vi "RUSHShoot.vi"(1 "In Cluster":T2) -> (0 "Out Cluster":T1)   [LabVIEW 2012]
panel:
  in  "Speed Multiplier":dbl=0.75
  in  "LinReg Adder":dbl=-0.5
  in  "LinReg Multiplier":dbl=0.01
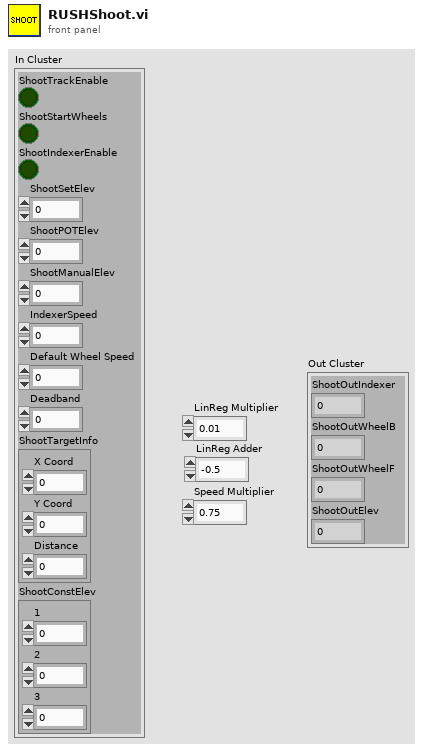
[diagram p1: front panel]
types:
  T1 = cluster{"ShootOutIndexer":dbl, "ShootOutWheelB":dbl, "ShootOutWheelF":dbl, "ShootOutElev":dbl}
  T2 = cluster{"ShootTrackEnable":bool, "ShootStartWheels":bool, "ShootIndexerEnable":bool, "ShootSetElev":dbl, "ShootPOTElev":dbl, "ShootManualElev":dbl, "IndexerSpeed":dbl, "Default Wheel Speed":dbl, "Deadband":dbl, "ShootTargetInfo":cluster{"X Coord":dbl, "Y Coord":dbl, "Distance":dbl}, "ShootConstElev":cluster{"1":dbl, "2":dbl, "3":dbl}}
  T3 = cluster{"X Coord":dbl, "Y Coord":dbl, "Distance":dbl}
  T4 = cluster{"ShootOutIndexer":dbl, "ShootOutWheelB":dbl, "ShootOutWheelF":dbl, "ShootManualElev":dbl}
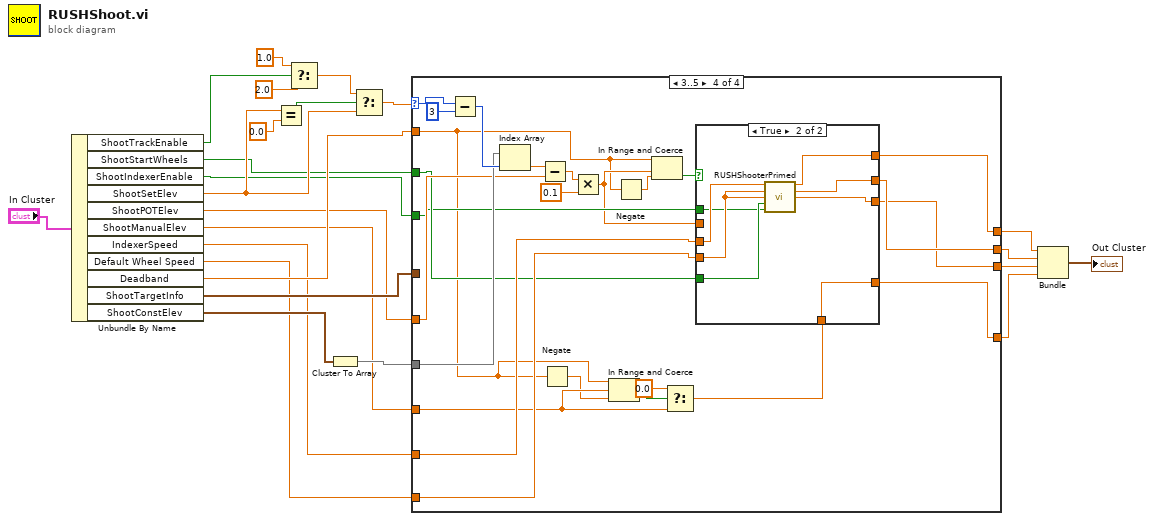
[diagram p0: block diagram]
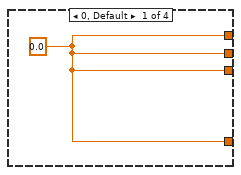
[diagram p2: hidden frame]
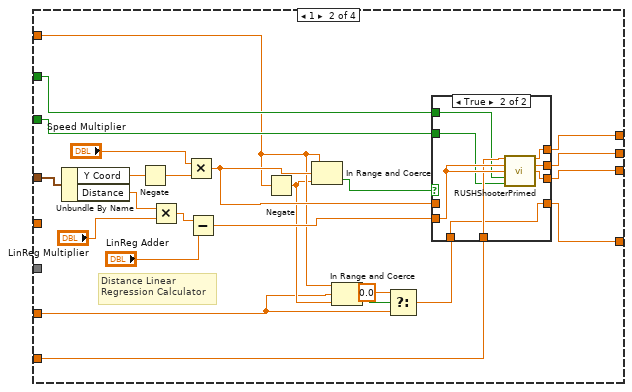
[diagram p3: hidden frame]
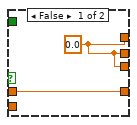
[diagram p4: hidden frame]
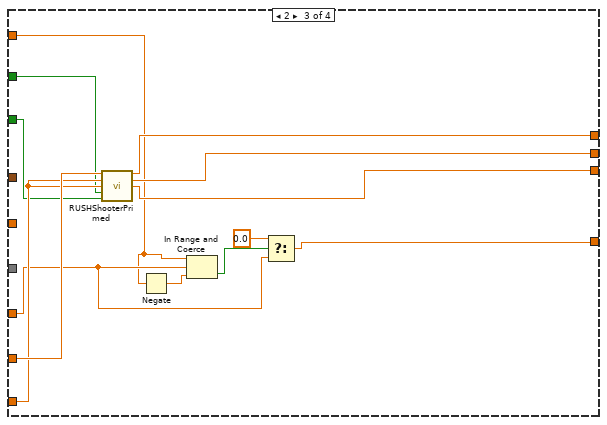
[diagram p5: hidden frame]
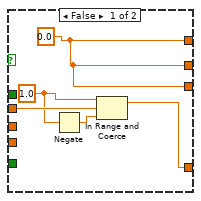
[diagram p6: hidden frame]
diagram:
  n1 = Unbundle By Name("In Cluster") -> ("ShootTrackEnable"=w16:bool, "ShootStartWheels"=w13:bool, "ShootIndexerEnable"=w12:bool, "ShootSetElev"=w15:dbl, "ShootPOTElev"=w10:dbl, "ShootManualElev"=w8:dbl, "IndexerSpeed"=w7:dbl, "Default Wheel Speed"=w6:dbl, "Deadband"=w14:dbl, "ShootTargetInfo"=w11:T3, "ShootConstElev"=w9:cluster{"1":dbl, "2":dbl, "3":dbl})
  n2 = Equal?(x=w15, y=0.0) -> (x = y?=w21:bool)
  n3 = Select(t=1.0, s=w16, f=2.0) -> (s? t:f=w20:dbl)
  n4 = Cluster To Array(cluster=w9) -> (array=w18:dbl[])
  n5 = Select(t=w20, s=w21, f=w15) -> (s? t:f=w19:dbl)
  n6 = case shown="3..5" w19 {
    selector: w19 -> [_ _ _ w97]
    tunnel: w13 -> [_ w44 w70 w83]
    tunnel: w12 -> [_ w43 w69 w82]
    tunnel: w11 -> [_ w49 _ _]
    tunnel: w10 -> [_ _ _ w92]
    tunnel: w18 -> [_ _ _ w94]
    tunnel: w8 -> [_ w27 w63 w75]
    tunnel: [w25 w37 w68 w89] -> w5
    tunnel: [w25 w36 w67 w88] -> w4
    tunnel: [w25 w35 w66 w87] -> w3
    tunnel: [w25 w33 w62 w86] -> w2
    tunnel: w7 -> [_ w32 w72 w85]
    tunnel: w6 -> [_ _ w71 w84]
    tunnel: w14 -> [_ w31 w61 w73]
    frame 0, Default {
      w25 = 0.0 ("ShootOutIndexer")
    }
    frame 1 {
      # "Distance Linear\nRegression Calculator"
      n7 = Unbundle By Name(w49) -> ("Y Coord"=w48:dbl, "Distance"=w42:dbl)
      n8 = Negate(x=w48) -> (-x=w47:dbl)
      n9 = Multiply(x=w42, y="LinReg Multiplier") -> (x*y=w40:dbl)
      n10 = Multiply(x="Speed Multiplier", y=w47) -> (x*y=w34:dbl)
      n11 = Subtract(x=w40, y="LinReg Adder") -> (x-y=w38:dbl)
      n12 = Negate(x=w31) -> (-x=w30:dbl)
      n13 = In Range and Coerce(upper limit=w31, x=w34, lower limit=w30) -> (In Range?=w45:bool)  [unwired: 1 out]
      n14 = In Range and Coerce(upper limit=w31, x=w27, lower limit=w30) -> (In Range?=w29:bool)  [unwired: 1 out]
      n15 = Select(t=0.0, s=w29, f=w27) -> (s? t:f=w26:dbl)
      n16 = case shown="True" w45 {
        tunnel: w44 -> [_ w53]
        tunnel: w43 -> [_ w54]
        tunnel: w38 -> [_ w59]
        tunnel: [w51 w58] -> w37
        tunnel: [w51 w57] -> w36
        tunnel: [w51 w56] -> w35
        tunnel: w34 -> [w50 _]
        tunnel: [w50 w52] -> w33
        tunnel: w32 -> [_ w55]
        tunnel: w26 -> [_ w52]
        frame False {
          w51 = 0.0 ("ShootOutIndexer")
        }
        frame True {
          n17 = call "RUSHShooterPrimed.vi"("IndexerSpeed"=w55, "WheelSpeedF"=w59, "WheelSpeedB"=w59, "ShootStartWheels"=w53, "ShootIndexerEnable"=w54) -> ("ShootOutIndexer"=w58:dbl, "ShootOutWheelB"=w57:dbl, "ShootOutWheelF"=w56:dbl)  [unwired: 8 in]
        }
      }
    }
    frame 2 {
      n18 = call "RUSHShooterPrimed.vi"("IndexerSpeed"=w72, "WheelSpeedF"=w71, "WheelSpeedB"=w71, "ShootStartWheels"=w70, "ShootIndexerEnable"=w69) -> ("ShootOutIndexer"=w68:dbl, "ShootOutWheelB"=w67:dbl, "ShootOutWheelF"=w66:dbl)  [unwired: 8 in]
      n19 = Negate(x=w61) -> (-x=w65:dbl)
      n20 = In Range and Coerce(upper limit=w61, x=w63, lower limit=w65) -> (In Range?=w64:bool)  [unwired: 1 out]
      n21 = Select(t=0.0, s=w64, f=w63) -> (s? t:f=w62:dbl)
    }
    frame 3..5 {
      n22 = Subtract(x=w97, y=3) -> (x-y=w95:i32)
      n23 = Index Array(array=w94, index=w95) -> (element=w93:dbl)
      n24 = Subtract(x=w93, y=w92) -> (x-y=w81:dbl)
      n25 = Negate(x=w73) -> (-x=w74:dbl)
      n26 = Multiply(x=w81, y=0.1) -> (x*y=w80:dbl)
      n27 = In Range and Coerce(upper limit=w73, x=w75, lower limit=w74) -> (In Range?=w78:bool)  [unwired: 1 out]
      n28 = Negate(x=w73) -> (-x=w91:dbl)
      n29 = In Range and Coerce(upper limit=w73, x=w80, lower limit=w91) -> (In Range?=w90:bool)  [unwired: 1 out]
      n30 = Select(t=0.0, s=w78, f=w75) -> (s? t:f=w76:dbl)
      n31 = case shown="True" w90 {
        tunnel: [w102 w106] -> w89
        tunnel: [w102 w105] -> w88
        tunnel: [w102 w104] -> w87
        tunnel: w80 -> [w101 _]
        tunnel: [w98 w103] -> w86
        tunnel: w85 -> [_ w110]
        tunnel: w84 -> [_ w109]
        tunnel: w83 -> [_ w108]
        tunnel: w82 -> [_ w107]
        tunnel: w76 -> [_ w103]
        frame False {
          w99 = 1.0 ("upper limit")
          w102 = 0.0
          n32 = Negate(x=w99) -> (-x=w100:dbl)
          n33 = In Range and Coerce(upper limit=w99, x=w101, lower limit=w100) -> (coerced(x)=w98:dbl)  [unwired: 1 out]
        }
        frame True {
          n34 = call "RUSHShooterPrimed.vi"("IndexerSpeed"=w110, "WheelSpeedF"=w109, "WheelSpeedB"=w109, "ShootStartWheels"=w108, "ShootIndexerEnable"=w107) -> ("ShootOutIndexer"=w106:dbl, "ShootOutWheelB"=w105:dbl, "ShootOutWheelF"=w104:dbl)  [unwired: 8 in]
        }
      }
    }
  }
  n35 = Bundle("ShootOutIndexer"=w5, "ShootOutWheelB"=w4, "ShootOutWheelF"=w3, "ShootManualElev"=w2) -> (→"Out Cluster":T4)  [unwired: 1 in]
